vi "ObtainRequestEvents.vi"(8 "ErrorArray In":errorcluster[](array[cluster]), 10 "CreateNew (F)":bool) -> (0 "ErrorArray Out":errorcluster[](array[cluster]), 2 "clRequestEvents":T1)   [LabVIEW 2014, in "Framework.lvlib"]
uses:
  Framework.lvlib
  Protected/Requests/clRequestEvents.ctl
  Protected/clUserEventType.ctl
  <userlib>/NIST/NISTErrorLib/NISTErrorLib.lvlib
panel:
  # "If you want to add other Request Events, open this typedef, copy an existing event and rename it to your event name."
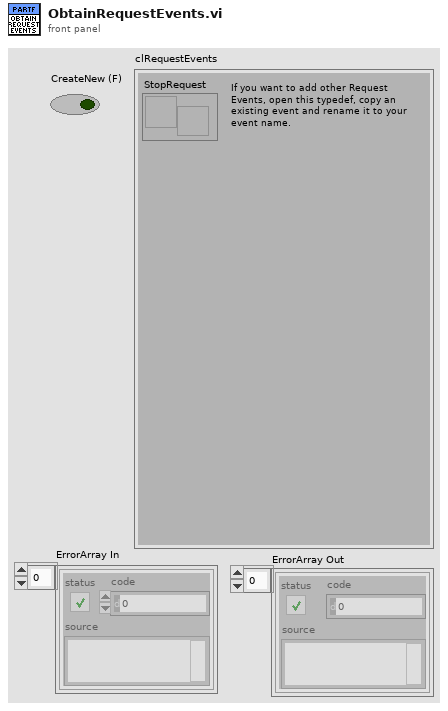
[diagram p1: front panel]
types:
  T1 = typedef "Framework.lvlib/clRequestEvents.ctl" = cluster{"StopRequest":refnum<user-event>}
  T2 = typedef "Framework.lvlib/clUserEventType.ctl" = cluster{"BusIndex":i8, "Data":variant}
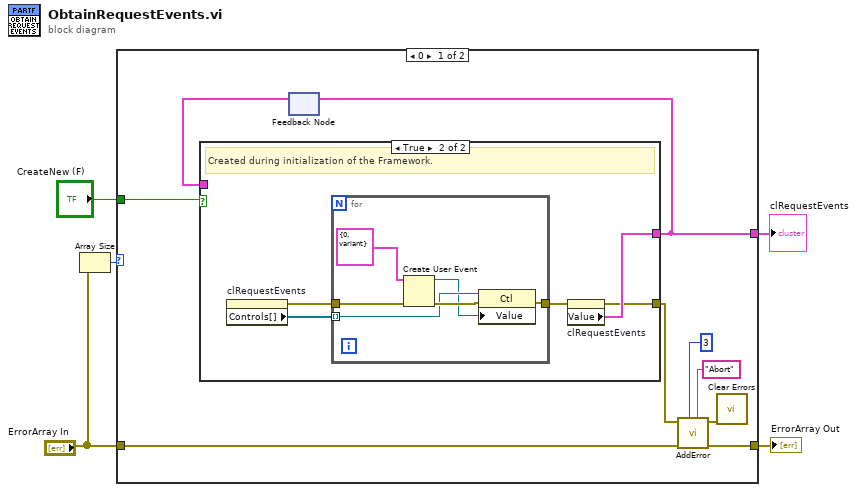
[diagram p0: block diagram]
diagram:
  n1 = Array Size(array="ErrorArray In") -> (size(s)=w3:i32)
  n2 = case shown="0" w3 {
    tunnel: "CreateNew (F)" -> [w14 _]
    tunnel: [w12 _] -> w4
    tunnel: "ErrorArray In" -> [w11 w27]
    tunnel: [w10 w27] -> w1
    frame 0 {
      n3 = feedback #1() -> (w13:T1)  [unwired: 1 in]
      n4 = case shown="True" w14 {
        tunnel: w13 -> [w15 _]
        tunnel: [_ w16] -> w6
        tunnel: [w15 w18] -> w12
        frame False {
        }
        frame True {
          # "Created during initialization of the Framework."
          n5 = property on="clRequestEvents" class="Clust (strict)"() -> (error out=w19:errorcluster, "Controls[]"=w20:refnum<vi>[])  [unwired: 2 in, 1 out]
          n6 = for {
            tunnel: w20 -> [w22] mode=indexing
            tunnel: w19 -> [w25]
            tunnel: [w23] -> w17
            n7 = Create User Event(user event datatype=T2 {"BusIndex"=0, "Data"=variant} ("clEventType"), error in=w25) -> (user event=w21:refnum<user-event>, error out=w24:errorcluster)
            n8 = property on="Property Node" class="Ctl"(reference=w22, error in=w24, "Value"=w21) -> (error out=w23:errorcluster)  [unwired: 1 out]
          }
          n9 = property on="clRequestEvents" class="Clust (strict)"(error in=w17) -> (error out=w16:errorcluster, "Value"=w18:T1)  [unwired: 1 in, 1 out]
        }
      }
      n10 = feedback-in #1(w12) -> ()
      n11 = call <userlib>:"AddError.vi"("Severity"="Abort" ("String"), "Priority"=u8 3, "ErrorArray"=w11, "error in (no error)"=w6) -> ("ErrorArray"=w10:errorcluster[], "error out"=w9:errorcluster)  [unwired: 6 in]
      n12 = call <vilib>:"Clear Errors.vi"("error in (no error)"=w9) -> ()  [unwired: 5 in, 2 out]
    }
    frame 1, Default {
    }
  }
  "clRequestEvents" <- w4
  "ErrorArray Out" <- w1
